vi "Write Test Sequence.vi"(10 "Test Sequence":T1, 11 "Toggle 6 in":refnum<class "Toggle 6.lvclass">) -> (3 "Toggle 6 out":refnum<class "Toggle 6.lvclass">)   [LabVIEW 2020, in "Toggle 6.lvclass"]
uses:
  Toggle 6.lvclass
  Controls/Test Sequence.ctl
  Controls/Register to Write.ctl
  Controls/EFuse modes enum.ctl
  Toggle 6.lvclass/Toggle 6.ctl
  PIC-device/PIC-Device.lvclass
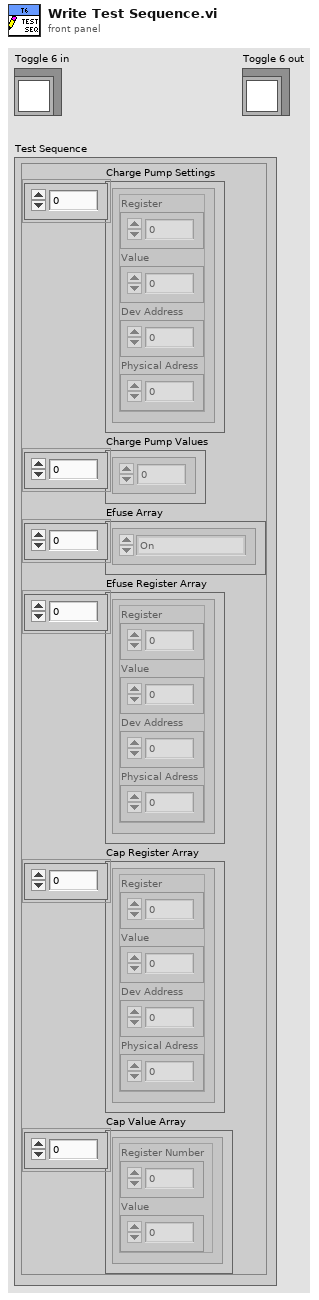
[diagram p1: front panel]
types:
  T1 = typedef "Toggle 6.lvclass/Test Sequence.ctl" = cluster{"Charge Pump Settings":T2[], "Charge Pump Values":dbl[], "Efuse Register Array":T2[], "Efuse Array":T3[], "Cap Register Array":T2[], "Cap Value Array":cluster{"Register Number":u32, "Value":dbl}[]}
  T2 = typedef "PIC-Device.lvclass/Register to Write.ctl" = cluster{"Register":u32, "Value":u32, "Dev Address":u32, "Physical Adress":u32}
  T3 = typedef "Toggle 6.lvclass/EFuse modes enum.ctl" = enum16{"On", "Off", "Both On and Off"}
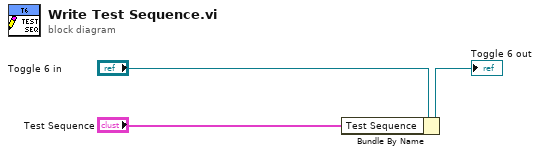
[diagram p0: block diagram]
diagram:
  n1 = Bundle By Name(cluster="Toggle 6 in", "Test Sequence"="Test Sequence") -> (→"Toggle 6 out":refnum<class "Toggle 6.lvclass">)
